vi "Module Loop.vi"(8 "error in (no error)":errorcluster, 11 "Role Manager in":refnum<class "Role Manager.lvclass">) -> (0 "error out":errorcluster, 3 "Role Manager out":refnum<class "Role Manager.lvclass">)   [LabVIEW 2020, in "Volatus.lvlib" / "Role Manager.lvclass"]
uses:
  Role Manager.lvclass
  C:/dev/lv20CE/relink/lv-volatus/Volatus/Module/Module.lvclass
  Module/Module.lvclass
  MessageQ/MessageQ.lvclass
  Role Manager.lvclass/Role Manager.ctl
  Module/Module.lvclass/Module.ctl
  MessageQ/MessageQ.lvclass/MessageQ.ctl
  Module/Send to Self.vi
  MessageQ/Send.vi
  <vilib>/Utility/error.llb/Error Cluster From Error Code.vi
  lv-promises/Promises/Promise/Promise.lvclass
  C:/dev/lv20CE/relink/lv-volatus/Volatus/Role Manager/Role Manager.lvclass
  Roles API/Roles API.lvclass
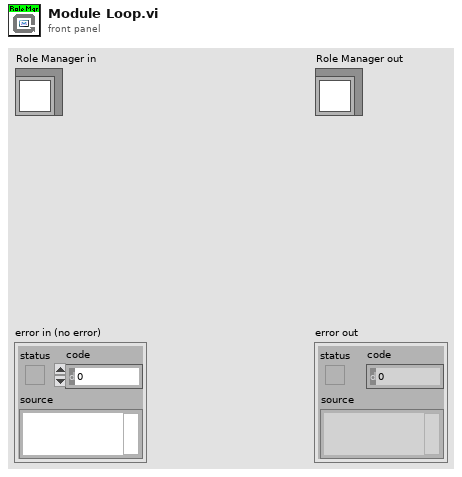
[diagram p1: front panel]
types:
  T1 = enum32{"Invalid", "Standard", "Closed", "Hidden", "Minimized", "Maximized"}
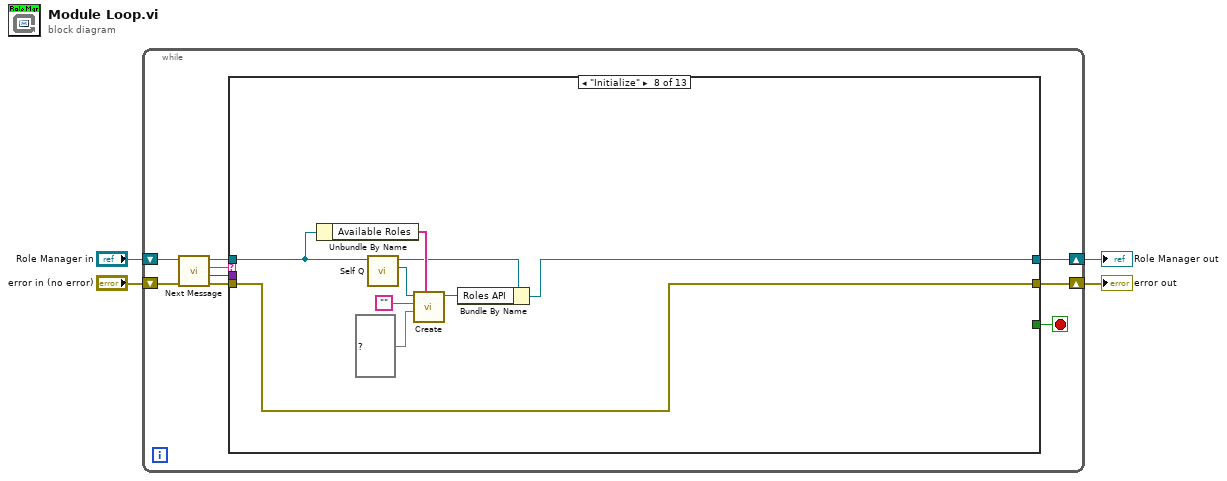
[diagram p0: block diagram]
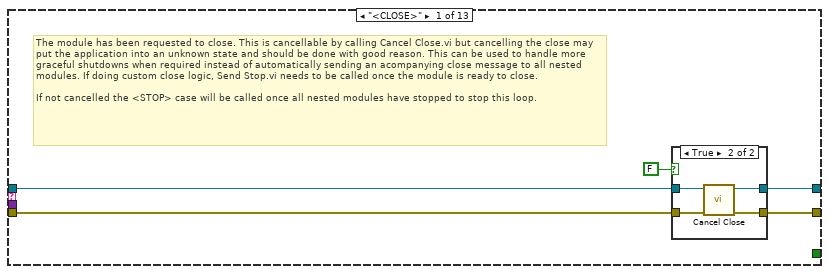
[diagram p2: hidden frame]
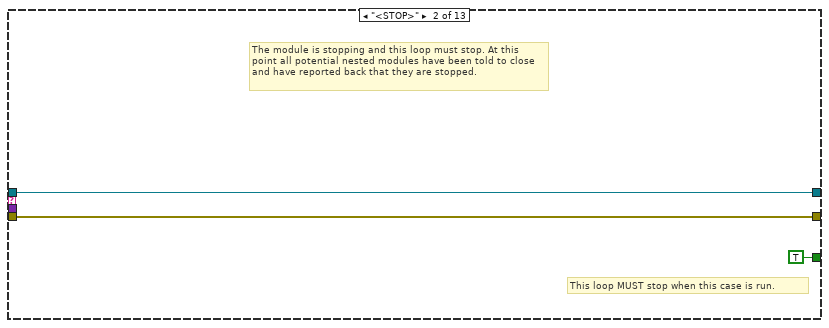
[diagram p4: hidden frame]
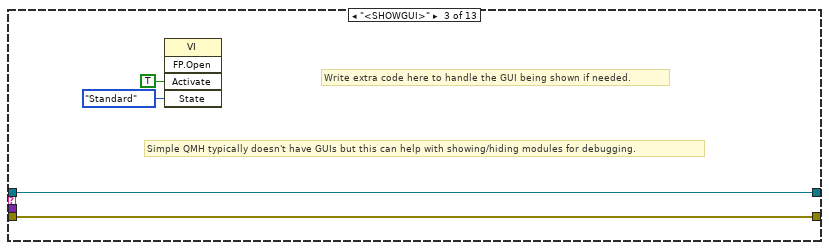
[diagram p5: hidden frame]
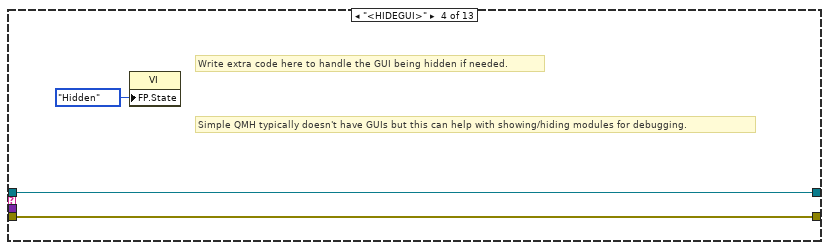
[diagram p6: hidden frame]
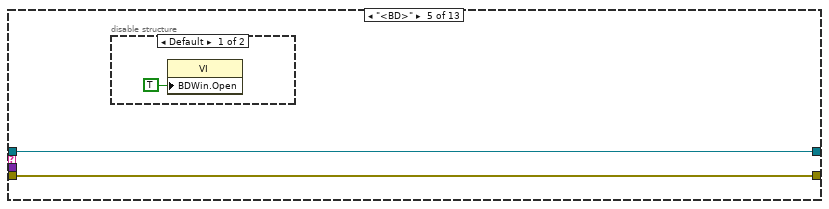
[diagram p7: hidden frame]
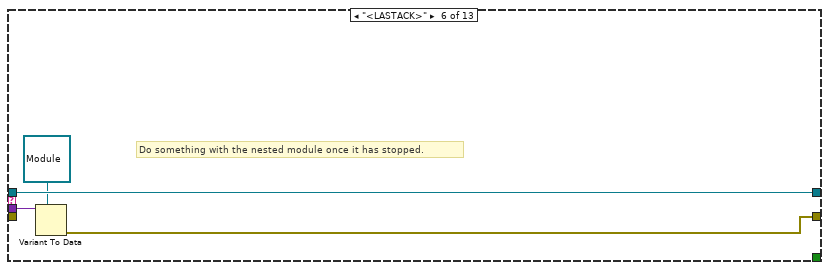
[diagram p9: hidden frame]
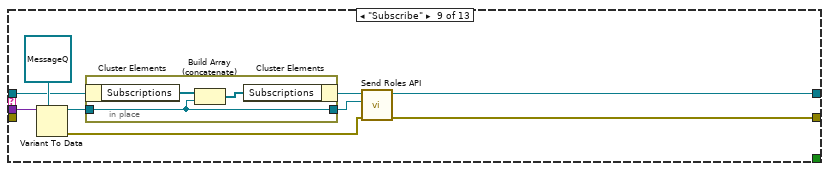
[diagram p11: hidden frame]
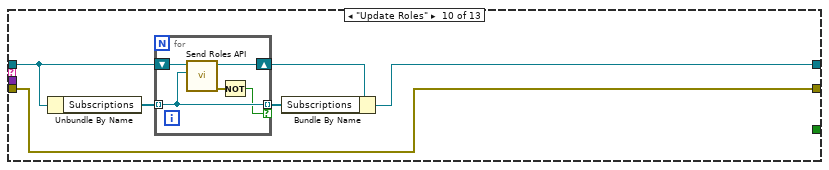
[diagram p12: hidden frame]
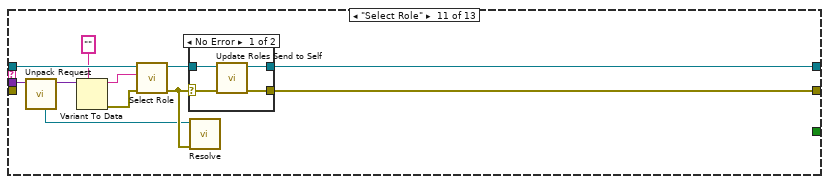
[diagram p13: hidden frame]
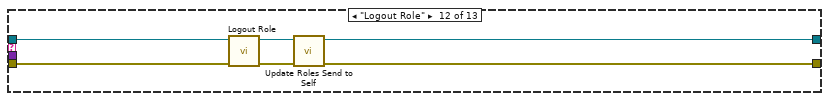
[diagram p15: hidden frame]
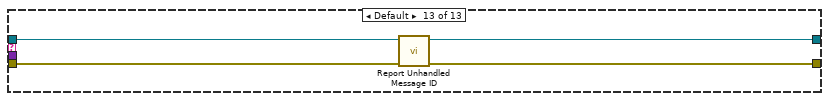
[diagram p16: hidden frame]
diagram:
  n1 = while {
    shift-right: [w8] -> w1
    shift-left: "Role Manager in" -> [w13]
    shift-right: [w5] -> w2
    shift-left: "error in (no error)" -> [w12]
    stop <- w7 stop-if-true
    n2 = call "Next Message.vi"("error in (no error)"=w12, "Module in"=w13) -> ("error out"=w11:errorcluster, "Data"=w6:variant, "ID"=w10:string, "Module out"=w9:refnum<class "Role Manager.lvclass">)  [unwired: 6 in]
    n3 = case shown="\"Initialize\"" w10 {
      tunnel: w11 -> [w18 w26 w30 w33 w35 _ w42 w44 _ w65 _ w98 w102]
      tunnel: w9 -> [w16 w27 w31 w34 w36 w41 w43 w49 w59 w69 w85 w96 w100]
      tunnel: [w15 w27 w31 w34 w36 w41 w43 w47 w53 w66 w76 w93 w99] -> w8
      tunnel: [_ TRUE _ _ _ _ _ _ _ _ _ _ _] -> w7
      tunnel: w6 -> [_ _ _ _ _ w40 _ _ w61 _ w83 _ _]
      tunnel: [w17 w26 w30 w33 w35 w38 w42 w44 w54 w65 w78 w95 w101] -> w5
      frame "<CLOSE>" {
        # "The module has been requested to close. This is cancellable by calling Cancel Close.vi but cancelling the close may put the application into an unknown state and should be done with good reason. This can be used to handle more graceful shutdowns when required instead of automatically sending an acompanying close message to all nested modules. If doing custom close logic, Send Stop.vi needs to be called once the module is ready to close.\n\nIf not cancelled the <STOP> case will be called once all nested modules have stopped to stop this loop."
        n4 = case shown="True" FALSE {
          tunnel: w18 -> [w19 w24]
          tunnel: [w19 w23] -> w17
          tunnel: w16 -> [w20 w22]
          tunnel: [w20 w21] -> w15
          frame False {
          }
          frame True {
            n5 = call "Cancel Close.vi"("error in (no error)"=w24, "Module in"=w22) -> ("error out"=w23:errorcluster, "Module out"=w21:refnum<class "Role Manager.lvclass">)  [unwired: 8 in]
          }
        }
      }
      frame "<STOP>" {
        # "This loop MUST stop when this case is run."
        # "The module is stopping and this loop must stop. At this point all potential nested modules have been told to close and have reported back that they are stopped."
      }
      frame "<SHOWGUI>" {
        # "Simple QMH typically doesn't have GUIs but this can help with showing/hiding modules for debugging."
        # "Write extra code here to handle the GUI being shown if needed."
        n6 = invoke class="VI" method="FP.Open"("Activate"=TRUE ("Activate?"), "State"=T1."Standard") -> ()  [unwired: 3 in, 5 out]
      }
      frame "<HIDEGUI>" {
        # "Simple QMH typically doesn't have GUIs but this can help with showing/hiding modules for debugging."
        # "Write extra code here to handle the GUI being hidden if needed."
        n7 = property class="VI"("FP.State"=T1."Hidden" ("Front Panel Window:State")) -> ()  [unwired: 2 in, 2 out]
      }
      frame "<BD>" {
        n8 = disable-structure shown="Default" {
          frame condition #0 (active) {
            n9 = property class="VI"("BDWin.Open"=TRUE ("Block Diagram Window:Open")) -> ()  [unwired: 2 in, 2 out]
          }
          frame condition #1 {
          }
        }
      }
      frame "<LASTACK>" {
        # "Do something with the nested module once it has stopped."
        n10 = Variant To Data(type=refnum<class "Module.lvclass"> refnum ("Volatus:Module"), Variant=w40) -> (error out=w38:errorcluster)  [unwired: 1 in, 1 out]
      }
      frame "<TIMEOUT>" {
        # "No message for this module was received in time"
      }
      frame "Initialize" {
        n11 = Unbundle By Name(w49) -> ("Available Roles"=w52:string[])
        n12 = call "Self Q.vi"("Module in"=w49) -> ("Self Q"=w51:refnum<class "MessageQ.lvclass">, "Module out"=w48:refnum<class "Role Manager.lvclass">)  [unwired: 9 in]
        n13 = call "Create.vi"("Available"=w52, "Effective Roles"=set{string} {}, "Current Role"="", "Manager"=w51) -> ("Roles API out"=w50:refnum<class "Roles API.lvclass">)  [unwired: 6 in, 1 out]
        n14 = Bundle By Name(cluster=w48, "Roles API"=w50) -> (w47:refnum<class "Role Manager.lvclass">)
      }
      frame "Subscribe" {
        n15 = Variant To Data(type=refnum<class "MessageQ.lvclass"> refnum ("Volatus:MessageQ"), Variant=w61) -> (data=w58:refnum<class "MessageQ.lvclass">, error out=w55:errorcluster)  [unwired: 1 in]
        n16 = in-place {
          in-place-border: w58 -> [w62]
          in-place-border: [w62] -> w56
          n17 = in-place-cluster #1(w59) -> ("Subscriptions"=w64:refnum<class "MessageQ.lvclass">[])
          n18 = Build Array (concatenate)(w64, w62) -> (w63:refnum<class "MessageQ.lvclass">[])
          n19 = in-place-cluster #1("Subscriptions"=w63) -> (w57:refnum<class "Role Manager.lvclass">)
        }
        n20 = call "Send Roles API.vi"("error in (no error)"=w55, "Subscriber"=w56, "Role Manager in"=w57) -> ("error out"=w54:errorcluster, "Role Manager out"=w53:refnum<class "Role Manager.lvclass">)  [unwired: 7 in]
      }
      frame "Update Roles" {
        n21 = Unbundle By Name(w69) -> ("Subscriptions"=w68:refnum<class "MessageQ.lvclass">[])
        n22 = for {
          shift-right: [w71] -> w70
          shift-left: w69 -> [w75]
          tunnel: w68 -> [w74] mode=indexing
          tunnel: [w74] -> w67 mode=indexing if=w72
          n23 = call "Send Roles API.vi"("Subscriber"=w74, "Role Manager in"=w75) -> ("error out"=w73:errorcluster, "Role Manager out"=w71:refnum<class "Role Manager.lvclass">)  [unwired: 8 in]
          n24 = Not(x=w73) -> (.not. x?=w72:bool)
        }
        n25 = Bundle By Name(cluster=w70, "Subscriptions"=w67) -> (w66:refnum<class "Role Manager.lvclass">)
      }
      frame "Select Role" {
        n26 = call "Unpack Request.vi"("Request Data"=w83) -> ("Data"=w82:variant, "Promise"=w79:refnum<class "Promise.lvclass">)  [unwired: 8 in, 1 out]
        n27 = Variant To Data(type="", Variant=w82) -> (data=w81:string, error out=w80:errorcluster)  [unwired: 1 in]
        n28 = call "Select Role.vi"("error in (no error)"=w80, "Role"=w81, "Role Manager in"=w85) -> ("error out"=w86:errorcluster, "Role Manager out"=w77:refnum<class "Role Manager.lvclass">)  [unwired: 7 in]
        n29 = case shown="No Error" w86 {
          selector: w86 -> [w90 w91]
          tunnel: [w89 w91] -> w78
          tunnel: w77 -> [w88 w92]
          tunnel: [w87 w92] -> w76
          frame No Error {
            n30 = call "Update Roles Send to Self.vi"("error in (no error)"=w90, "Role Manager in"=w88) -> ("error out"=w89:errorcluster, "Role Manager out"=w87:refnum<class "Role Manager.lvclass">)  [unwired: 8 in]
          }
          frame Error {
          }
        }
        n31 = call "Resolve.vi"("error in (no error)"=w86, "Promise in"=w79) -> ()  [unwired: 8 in, 2 out]
      }
      frame "Logout Role" {
        n32 = call "Logout Role.vi"("error in (no error)"=w98, "Role Manager in"=w96) -> ("error out"=w97:errorcluster, "Role Manager out"=w94:refnum<class "Role Manager.lvclass">)  [unwired: 8 in]
        n33 = call "Update Roles Send to Self.vi"("error in (no error)"=w97, "Role Manager in"=w94) -> ("error out"=w95:errorcluster, "Role Manager out"=w93:refnum<class "Role Manager.lvclass">)  [unwired: 8 in]
      }
      frame Default {
        n34 = call "Report Unhandled Message ID.vi"("error in (no error)"=w102, "Module in"=w100) -> ("error out"=w101:errorcluster, "Module out"=w99:refnum<class "Role Manager.lvclass">)  [unwired: 8 in]
      }
    }
  }
  "error out" <- w2
  "Role Manager out" <- w1
